vi "Wyznaczenie azymutu jaki należy obrać by dotrzeć do zadanego punktu.vi"(10 "Położenie końcowe":cluster{"X":dbl, "Y":dbl}, 11 "Położenie aktualne":cluster{"X":dbl, "Y":dbl}) -> (3 "Azymut":dbl)   [LabVIEW 2015, in "Biblioteka moduł map v3.lvlib" / "Matematyczne.lvlib"]
uses:
  Matematyczne.lvlib
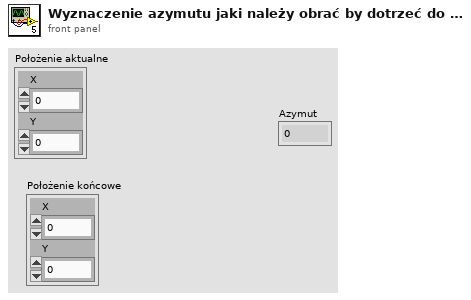
[diagram p1: front panel]
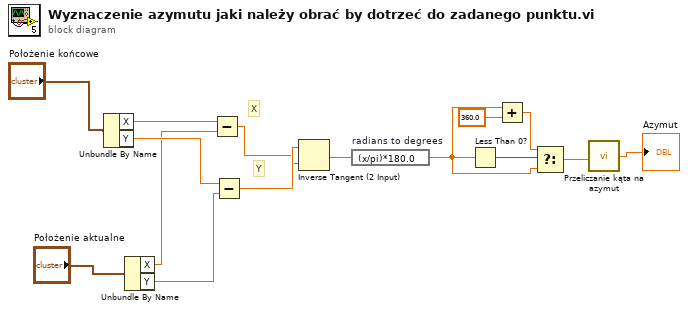
[diagram p0: block diagram]
diagram:
  # "Y"
  # "X"
  n1 = Unbundle By Name("Położenie końcowe") -> ("X"=w12:dbl, "Y"=w11:dbl)
  n2 = Unbundle By Name("Położenie aktualne") -> ("X"=w10:dbl, "Y"=w9:dbl)
  n3 = Subtract(x=w12, y=w10) -> (x-y=w7:dbl)
  n4 = Subtract(x=w11, y=w9) -> (x-y=w8:dbl)
  n5 = Inverse Tangent (2 Input)(1:w7, 2:w8) -> (0:w6:dbl)
  n6 = expression code="(x/pi)*180.0" "radians to degrees"(w6) -> (w4:dbl)
  n7 = Less Than 0?(x=w4) -> (x < 0?=w5:bool)
  n8 = Add(x=w4, y=360.0) -> (x+y=w2:dbl)
  n9 = Select(t=w2, s=w5, f=w4) -> (s? t:f=w1:dbl)
  n10 = call "Przeliczanie kąta na azymut.vi"("Kąt [stoponie]"=w1) -> ("Azymut [stopnie]"=→"Azymut":dbl)  [unwired: 4 in]
